vi "Write Message.vi"(0 "SRL Data":u8[][](array[numeric]) format="%.0x", 1 "Wait Ticks":u32, 5 "Socket Mask":u32=1 format="%06x", 7 "Cycle Mode":bool, 11 "error in":errorcluster, 14 "FPGA":T1) -> (8 "Status":u8[](array[numeric]), 15 "error out":errorcluster)   [LabVIEW 2017, in "Host SRL.lvlib"]
uses:
  Host SRL.lvlib
  Type Defs/WSVCAP SHL FPGA Enum.ctl
  Type Defs/WSVCAP SHL Top Level Write Read State Enum.ctl
  Type Defs/WSVCAP SHL State.ctl
  Type Defs/WSVCAP SHL Top Level Control Enum.ctl
  Type Defs/WSVCAP SHL Transaction Enum.ctl
panel:
  out "Write Data":u64[](array[numeric]) format="%032b"
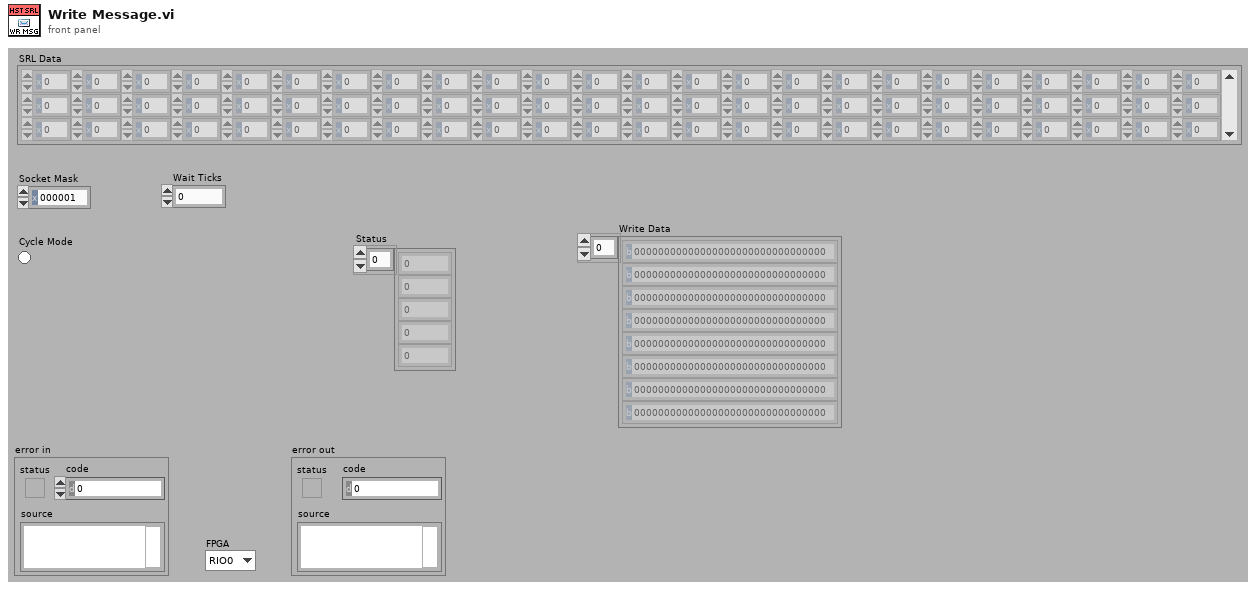
[diagram p1: front panel]
types:
  T1 = typedef "WSVCAP SHL FPGA Enum.ctl" = enum16{"RIO0", "RIO1"}
  T2 = typedef "WSVCAP SHL Top Level Write Read State Enum.ctl" = enum16{"Start", "Write", "Read", "Get Status", "Wait Until Done"}
  T3 = typedef "WSVCAP SHL State.ctl" = enum8{"Idle", "Transfer Data"}
  T4 = typedef "WSVCAP SHL Transaction Enum.ctl" = enum16{"I2C-Read Data", "I2C-Write Data", "RFFE-Ext Write", "RFFE-Ext Read", "SRL-Write Data"}
  T5 = typedef "WSVCAP SHL Top Level Control Enum.ctl" = enum16{"Start", "Cmd", "Transaction", "Wait Ticks", "Socket Mask", "UUT Set", "Slave Address", "Sub Address", "Bytes to Write", "Bytes to Read", "Write Data", "Write Flag", "Read Data", "Read Flag", "Ack Read", "Read Status Flag", "Ack Read Status", "Status", "Cycle Count", "Stop Cycle", "Exit"}
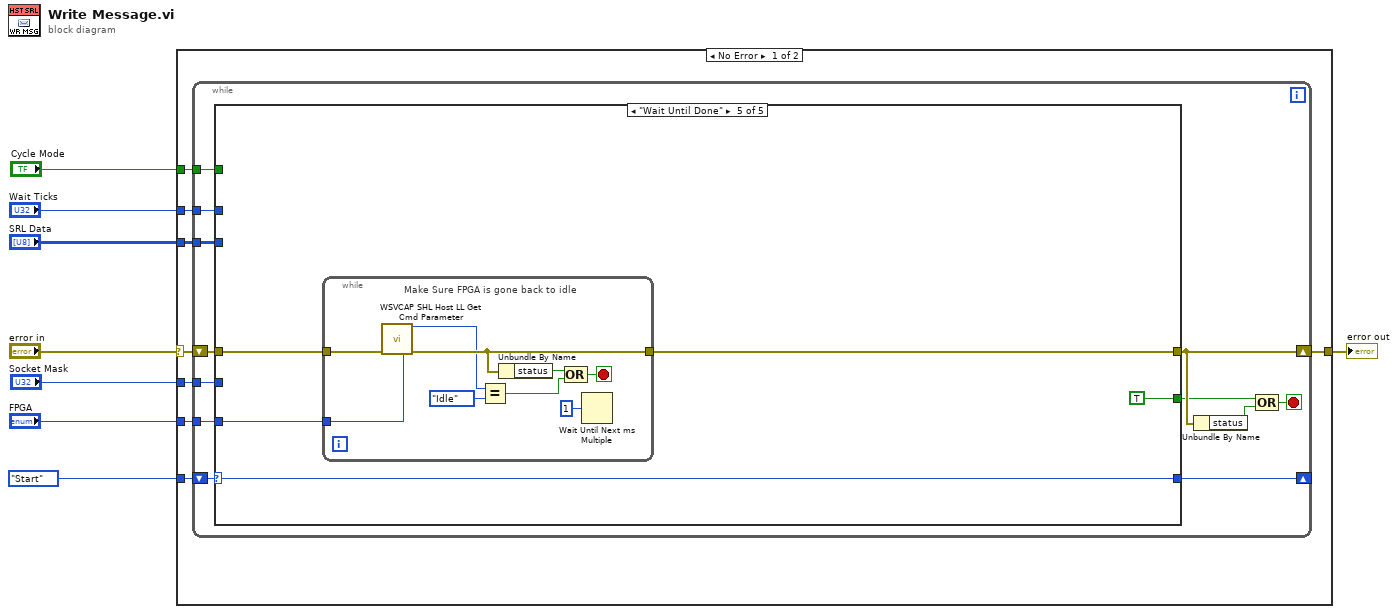
[diagram p0: block diagram]
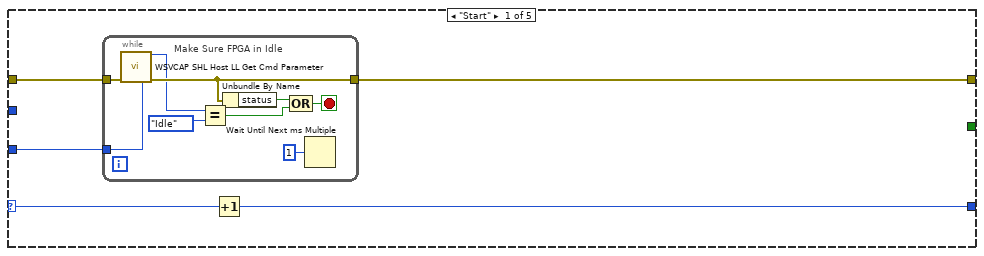
[diagram p2: hidden frame]
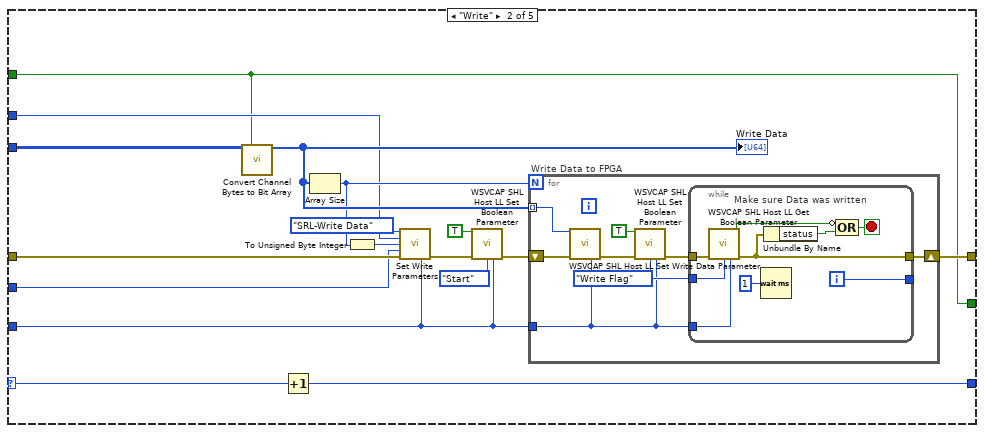
[diagram p3: hidden frame]
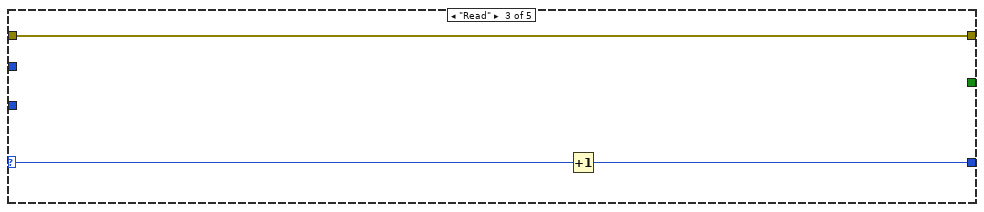
[diagram p4: hidden frame]
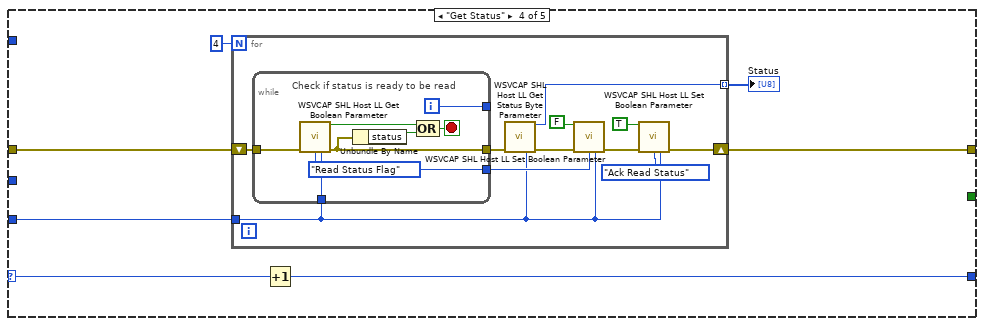
[diagram p5: hidden frame]
diagram:
  n1 = case shown="No Error" "error in" {
    selector: "error in" -> [w12 w120]
    tunnel: [w16 w120] -> w8
    tunnel: WSVCAP_SHL_Top_Level_Write_Read_State_Enum."Start" ("Write Read State") -> [w15 _]
    tunnel: "SRL Data" -> [w14 _]
    tunnel: "Socket Mask" -> [w13 _]
    tunnel: "Wait Ticks" -> [w11 _]
    tunnel: "FPGA" -> [w10 _]
    tunnel: "Cycle Mode" -> [w9 _]
    frame No Error {
      n2 = while {
        shift-right: [w27] -> w16
        shift-left: w12 -> [w28]
        shift-right: [w22] -> _
        shift-left: w15 -> [w23]
        tunnel: w14 -> [w21]
        tunnel: w13 -> [w20]
        tunnel: w11 -> [w19]
        tunnel: w10 -> [w18]
        tunnel: w9 -> [w17]
        stop <- w24 stop-if-true
        n3 = case shown="\"Wait Until Done\"" w23 {
          selector: w23 -> [w32 w58 w79 w84 w108]
          tunnel: w28 -> [w33 w51 w77 w86 w110]
          tunnel: [w30 w59 w77 w85 w109] -> w27
          tunnel: [_ w43 _ _ TRUE] -> w26
          tunnel: [w31 w56 w78 w83 w108] -> w22
          tunnel: w21 -> [_ w47 _ _ _]
          tunnel: w20 -> [_ w48 _ _ _]
          tunnel: w19 -> [_ w46 _ _ _]
          tunnel: w18 -> [w29 w44 _ w80 w106]
          tunnel: w17 -> [_ w43 _ _ _]
          frame "Start" {
            n4 = while {
              tunnel: w33 -> [w38]
              tunnel: [w37] -> w30
              tunnel: w29 -> [w34]
              stop <- w42 stop-if-true
              # "Make Sure FPGA in Idle"
              n5 = call "WSVCAP SHL Host LL Get Cmd Parameter.vi"("error in (no error)"=w38, "FPGA"=w34) -> ("I2C_Cmd"=w36:T3, "error out"=w37:errorcluster)  [unwired: 12 in]
              n6 = Equal?(x=w36, y=WSVCAP_SHL_State."Idle" ("Type")) -> (x = y?=w40:bool)
              n7 = Unbundle By Name(w37) -> ("status"=w35:bool)
              n8 = Compound Arithmetic op=OR(w35, w40) -> (w42:bool)
              n9 = Wait Until Next ms Multiple(millisecond multiple=u32 1) -> ()  [unwired: 1 out]
            }
            n10 = Increment(x=w32) -> (x+1=w31:T2)
          }
          frame "Write" {
            # "Write Data to FPGA"
            n11 = call "Convert Channel Bytes to Bit Array.vi"("SRL Data"=w47, "Cycle Mode In"=w43) -> ("Write Data"=w57:u64[])  [unwired: 13 in]
            "Write Data" <- w57
            n12 = Increment(x=w58) -> (x+1=w56:T2)
            n13 = Array Size(array=w57) -> (size(s)=w49:i32)
            n14 = To Unsigned Byte Integer(number=w49) -> (unsigned 8bit integer=w52:u8)
            n15 = call "Set Write Parameters.vi"("Transaction"=WSVCAP_SHL_Transaction_Enum."SRL-Write Data", "Wait Ticks"=w46, "Bytes to Write"=w52, "Socket Mask [U32]"=w48, "error in (no error)"=w51, "FPGA"=w44) -> ("error out"=w55:errorcluster)  [unwired: 9 in]
            n16 = call "WSVCAP SHL Host LL Set Boolean Parameter.vi"("Boolean In"=TRUE, "error in (no error)"=w55, "FPGA Top Level Control"=WSVCAP_SHL_Top_Level_Control_Enum."Start", "FPGA"=w44) -> ("error out"=w50:errorcluster)  [unwired: 11 in]
            n17 = for {
              N: w49 -> [_]
              shift-right: [w67] -> w59
              shift-left: w50 -> [w66]
              tunnel: w57 -> [w65] mode=indexing
              tunnel: w44 -> [w60]
              w61 = WSVCAP_SHL_Top_Level_Control_Enum."Write Flag" ("FPGA Top Level Control")
              n18 = call "WSVCAP SHL Host LL Set Write Data Parameter.vi"("Write Byte In"=w65, "error in (no error)"=w66, "FPGA"=w60) -> ("error out"=w64:errorcluster)  [unwired: 12 in]
              n19 = call "WSVCAP SHL Host LL Set Boolean Parameter.vi"("Boolean In"=TRUE, "error in (no error)"=w64, "FPGA Top Level Control"=w61, "FPGA"=w60) -> ("error out"=w62:errorcluster)  [unwired: 11 in]
              n20 = while {
                tunnel: w62 -> [w74]
                tunnel: [w73] -> w67
                tunnel: w61 -> [w71]
                tunnel: [w69] -> _
                tunnel: w60 -> [w68]
                i -> [w69]
                stop <- w76 stop-if-true
                # "Make sure Data was written"
                n21 = call "WSVCAP SHL Host LL Get Boolean Parameter.vi"("error in (no error)"=w74, "FPGA Top Level Control"=w71, "FPGA"=w68) -> ("Boolean Out"=w72:bool, "error out"=w73:errorcluster)  [unwired: 11 in]
                n22 = Wait (ms)(milliseconds to wait=u32 1) -> ()  [unwired: 1 out]
                n23 = Unbundle By Name(w73) -> ("status"=w70:bool)
                n24 = Compound Arithmetic op=OR(invert w72, w70) -> (w76:bool)
              }
            }
          }
          frame "Read" {
            n25 = Increment(x=w79) -> (x+1=w78:T2)
          }
          frame "Get Status" {
            n26 = for {
              N: 4 -> [_]
              shift-right: [w96] -> w85
              shift-left: w86 -> [w97]
              tunnel: [w88] -> w81 mode=indexing
              tunnel: w80 -> [w87]
              n27 = while {
                tunnel: w97 -> [w103]
                tunnel: [w102] -> w95
                tunnel: [w100] -> w93
                tunnel: [w99] -> _
                tunnel: w87 -> [w98]
                i -> [w99]
                stop <- w105 stop-if-true
                w100 = WSVCAP_SHL_Top_Level_Control_Enum."Read Status Flag" ("FPGA Top Level Control")
                # "Check if status is ready to be read"
                n28 = call "WSVCAP SHL Host LL Get Boolean Parameter.vi"("error in (no error)"=w103, "FPGA Top Level Control"=w100, "FPGA"=w98) -> ("Boolean Out"=w104:bool, "error out"=w102:errorcluster)  [unwired: 11 in]
                n29 = Unbundle By Name(w102) -> ("status"=w101:bool)
                n30 = Compound Arithmetic op=OR(w104, w101) -> (w105:bool)
              }
              n31 = call "WSVCAP SHL Host LL Get Status Byte Parameter.vi"("error in (no error)"=w95, "FPGA"=w87) -> ("I2C Status Byte"=w88:u8, "error out"=w94:errorcluster)  [unwired: 12 in]
              n32 = call "WSVCAP SHL Host LL Set Boolean Parameter.vi"("Boolean In"=FALSE ("Read Flag"), "error in (no error)"=w94, "FPGA Top Level Control"=w93, "FPGA"=w87) -> ("error out"=w89:errorcluster)  [unwired: 11 in]
              n33 = call "WSVCAP SHL Host LL Set Boolean Parameter.vi"("Boolean In"=TRUE ("Write Flag"), "error in (no error)"=w89, "FPGA Top Level Control"=WSVCAP_SHL_Top_Level_Control_Enum."Ack Read Status", "FPGA"=w87) -> ("error out"=w96:errorcluster)  [unwired: 11 in]
            }
            "Status" <- w81
            n34 = Increment(x=w84) -> (x+1=w83:T2)
          }
          frame "Wait Until Done" {
            n35 = while {
              tunnel: w110 -> [w114]
              tunnel: [w113] -> w109
              tunnel: w106 -> [w111]
              stop <- w116 stop-if-true
              # "Make Sure FPGA is gone back to idle"
              n36 = call "WSVCAP SHL Host LL Get Cmd Parameter.vi"("error in (no error)"=w114, "FPGA"=w111) -> ("I2C_Cmd"=w112:T3, "error out"=w113:errorcluster)  [unwired: 12 in]
              n37 = Equal?(x=w112, y=WSVCAP_SHL_State."Idle") -> (x = y?=w117:bool)
              n38 = Unbundle By Name(w113) -> ("status"=w118:bool)
              n39 = Compound Arithmetic op=OR(w118, w117) -> (w116:bool)
              n40 = Wait Until Next ms Multiple(millisecond multiple=u32 1) -> ()  [unwired: 1 out]
            }
          }
        }
        n41 = Unbundle By Name(w27) -> ("status"=w25:bool)
        n42 = Compound Arithmetic op=OR(w26, w25) -> (w24:bool)
      }
    }
    frame Error {
    }
  }
  "error out" <- w8
